vi "Robot Global Data.vi"() -> ()   [LabVIEW 2011]
doc: "This global VI can contain as many global variables as you need. Place a control on the panel, give it a good name. To read or write to it from a VI, drag the icon to the diagram of that VI. You can also drag from the project. Click on the node to change which global you access. You shouldn't have multiple locations writing to a global or it will cause a race-condition."
uses:
  <vilib>/Rock Robotics/WPI/Camera/WPI_CameraImageSize.ctl
panel:
  in  "Camera Settings":T2={"fps"=15, "compression"=30, "Image Size"=enum."160x120"}
  in  "Camera IP":string="10.0.27.11"
  out "Auton Index":dbl
  out "Auton Dist Travelled":dbl
  out "Robot Angle 2":dbl
  in  "pasco_point_slider":dbl(slide) scale=0.0..10.0
  out "GlobalVariableArray":cluster{"name":string, "va;":dbl}[](array[cluster])=[{"name"="Val1", "va;"=1.0}, {"name"="Val2", "va;"=2.0}, {"name"="Val3", "va;"=3.0}, {"name"="Val4", "va;"=4.0}]
  out "Light_On":bool=TRUE
  out "file_read_error":bool
  in  "file_read_test_5":dbl
  in  "file_read_test_4":dbl
  in  "file_read_test_3":dbl
  in  "file_read_test_2":dbl
  in  "file_read_test_1":dbl
  in  "YStart":dbl
  in  "XStart":dbl
  in  "AutonMode":u32
  out "VisitedEnabled":bool
  out "AutonEnabled":bool
  out "RobotEnabled":bool
  in  "CurrentAutonFile":string
  out "AutonArray":dbl[][](array[numeric])
  in  "AutonFiles":string[](array[string])
  in  "NumberOfAutonFiles":dbl
  in  "LeftShifter_Pos":dbl
  in  "RightShifter_Pos":dbl
  in  "Forward Ultrasonic":dbl
  in  "Minibot Trigger":bool
  out "Robot Angle":dbl
  out "Left Drive Rate":dbl
  out "Right Drive Rate":dbl
  in  "Arduino Setpoint":string="1"
  in  "Arduino Right":dbl
  in  "Arduino Left":dbl
  in  "Autonomous":bool
  out "PWM 1(Left Drive)":dbl
  out "PWM 2(Right Drive)":dbl
  out "Arm Integral Reset":bool
  out "Initialize Setpoint":bool=TRUE
  out "Dashboard DI 4":bool
  out "Auton Switch 2":bool
  out "Auton Switch 1":bool
  in  "Auto Move":bool
  out "Right Drive Distance":dbl
  out "Left Drive Distance":dbl
  out "Dashboard DI 3":bool
  out "Dashboard DI 1":bool=TRUE
  in  "Tube Release State":dbl
  out "Joystick VS. Control Pad":bool
  out "Right Drive Output":dbl
  out "Left Drive Output":dbl
  in  "AI 7 Setpoint":dbl
  in  "AI 5 Setpoint":dbl
  out "Joystick 2":T3
  out "Joystick 1":T3
  out "Joystick 4":T3
  out "Joystick 3":T3
  in  "LED toggle rate (ms)":u32
  in  "Enable Vision":bool
  # "Vision"
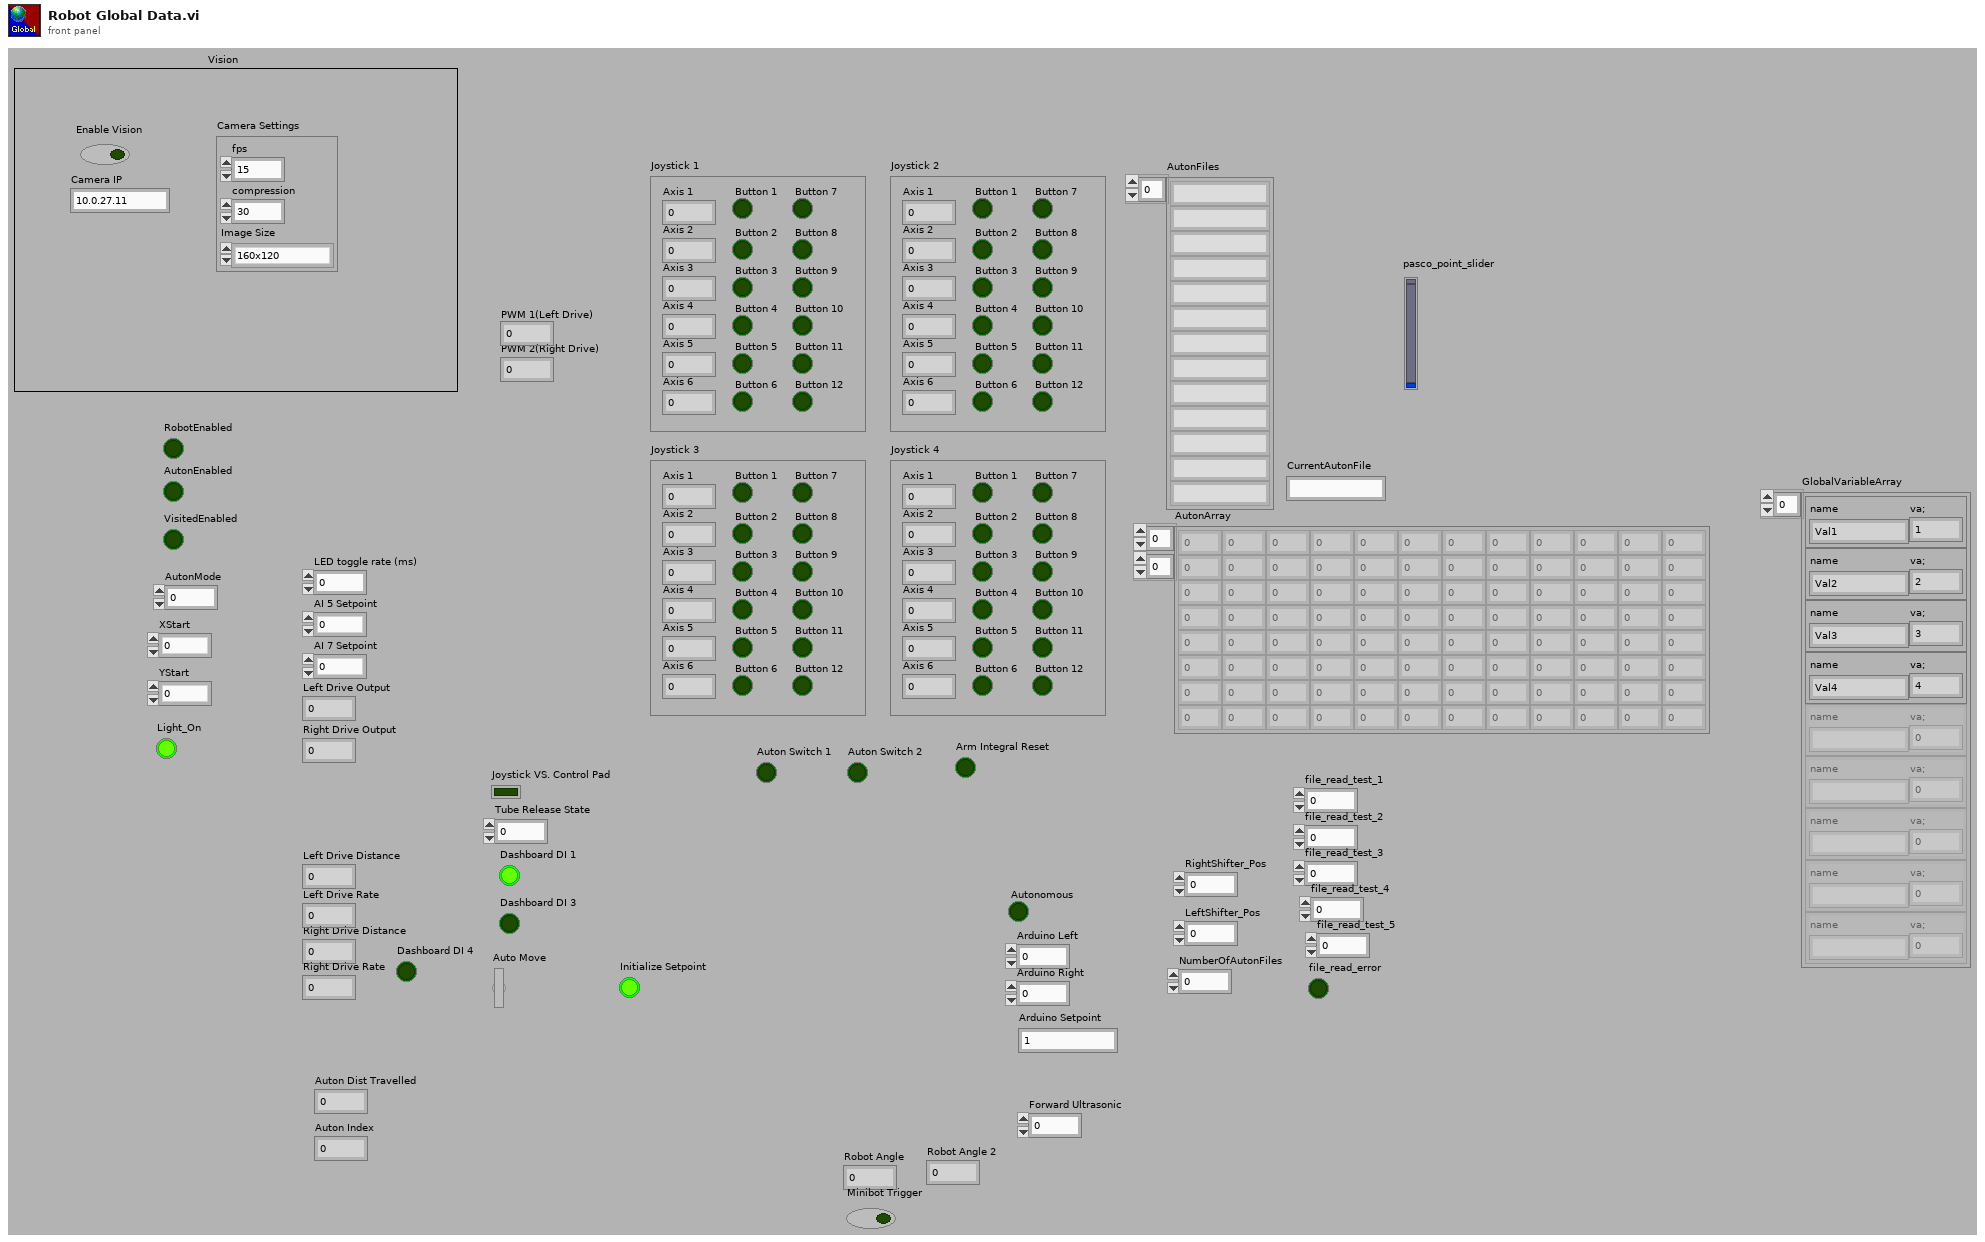
[diagram p1: front panel]
types:
  T1 = typedef "WPI_CameraImageSize.ctl" = enum16{"640x480", "320x240", "160x120"}
  T2 = cluster{"fps":i32, "compression":i32, "Image Size":T1}
  T3 = cluster{"Axis 1":dbl, "Axis 2":dbl, "Axis 3":dbl, "Axis 4":dbl, "Axis 5":dbl, "Axis 6":dbl, "Button 1":bool, "Button 2":bool, "Button 3":bool, "Button 4":bool, "Button 5":bool, "Button 6":bool, "Button 7":bool, "Button 8":bool, "Button 9":bool, "Button 10":bool, "Button 11":bool, "Button 12":bool}
diagram:
